vi "禹山电导率_获取温度和测量值.vi"(8 "error in (no error)":errorcluster caption="错误输入（无错误）", 11 "MB session in":refnum<class "MB_Master.lvclass">) -> (0 "error out":errorcluster caption="错误输出", 2 "输出值":cluster{"温度测量值":sgl, "电导率":sgl, "错误标志":u16} {"错误标志" items=["NO Error"=0, "量程切换错误标识"=255]}, 3 "MB session out":refnum<class "MB_Master.lvclass">)   [LabVIEW 2016, in "斯坦道多参数.lvlib"]
uses:
  <vilib>/Plasmionique/MB Master/MB_Master/MB_Master.lvclass
  <vilib>/Plasmionique/MB Master/MB Master.lvlib
  <vilib>/ptbypt/NI_PtbyPt.lvlib
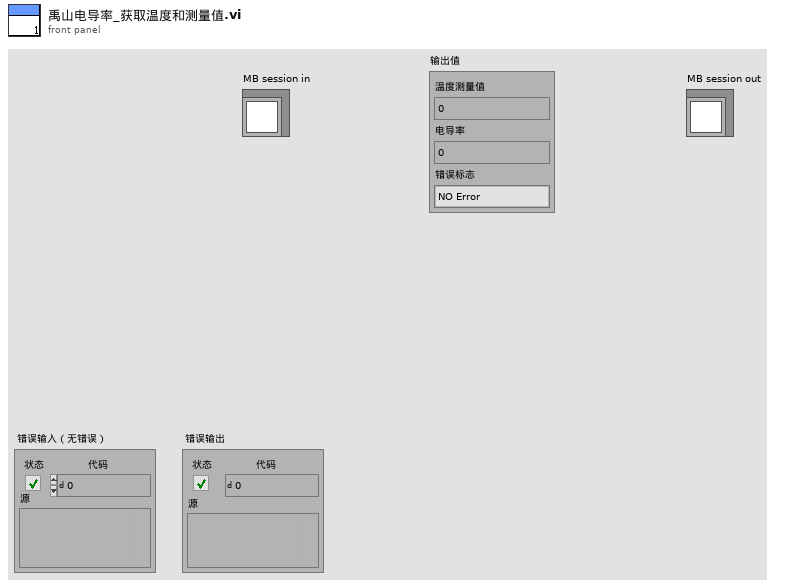
[diagram p1: front panel]
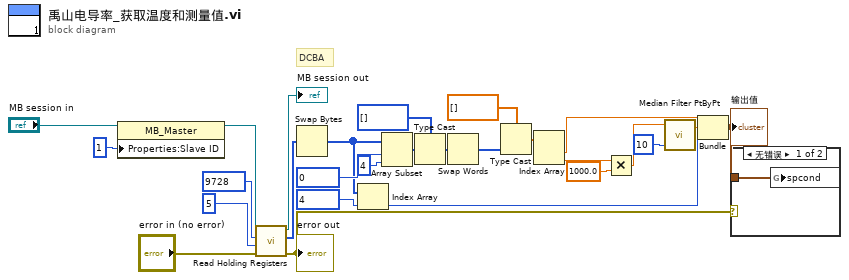
[diagram p0: block diagram]
diagram:
  # "DCBA"
  n1 = property class="MB_Master"(reference="MB session in", "Properties:Slave ID"=u16 1 ("y")) -> (reference out=w19:refnum<class "MB_Master.lvclass">)  [unwired: 1 in, 1 out]
  n2 = call <vilib>:"Read Holding Registers.vi"("error in (no error)"="error in (no error)", "quantity"=u16 5, "starting address"=u16 9728, "MB session in"=w19) -> ("error out"=w13:errorcluster, "Registers"=w17:u16[], "MB session out"=→"MB session out":refnum<class "MB_Master.lvclass">)  [unwired: 5 in]
  "error out" <- w13
  n3 = Swap Bytes(anything=w17) -> (byte swapped=w7:u16[])
  n4 = Index Array(array=w7, index=u16 4 ("starting address")) -> (element=w6:u16)
  n5 = Array Subset(array=w7, index=u16 0 ("starting address"), length=4 ("长度")) -> (w11:u16[])
  n6 = Type Cast(type=u32[] [] ("数组 2"), x=w11) -> (*(type *) &x=w23:u32[])
  n7 = Swap Words(1:w23) -> (0:w25:u32[])
  n8 = Type Cast(type=sgl[] [] ("数组 2"), x=w25) -> (*(type *) &x=w21:sgl[])
  n9 = Index Array(array=w21) -> (element #1=w16:sgl, element #2=w15:sgl)  [unwired: 2 in]
  n10 = Multiply(x=w15, y=sgl 1000.0) -> (x*y=w2:sgl)
  n11 = call <vilib>:"Median Filter PtByPt.vi"("rank"=10, "x"=w2) -> ("Filtered x"=w1:dbl)  [unwired: 2 in, 1 out]
  n12 = Bundle("数值"=w16, "Filtered x"=w1, w6) -> (w12:cluster{"数值":sgl, "Filtered x":dbl, u16})  [unwired: 1 in]
  "输出值" <- w12
  n13 = case shown="无错误" w13 {
    tunnel: w12 -> [w28 _]
    frame No Error {
      n14 = global write "禹山过程全局变量.vi" "spcond"(w28) -> ()
    }
    frame Error {
    }
  }
